vi "WriteExternalInterfaces.vi"(8 "Error In":errorcluster, 10 "ExternalInterfaces":T1[](array[typedef]), 11 "OpenCVCam in":refnum<class "OpenCVCam.lvclass">) -> (0 "Error Out":errorcluster, 3 "OpenCVCam out":refnum<class "OpenCVCam.lvclass">)   [LabVIEW 2021, in "OpenCVCam.lvclass"]
uses:
  OpenCVCam.lvclass
  .Externals/Library_TAF_Support/ClusterArrayConversion/BundledArray.ctl
  OpenCVCam.lvclass/OpenCVCam.ctl
  0f9fbe56-9f9a-4601-8b43-1fc07a995cee.vi
  0f9fbe56-9f9a-4601-8b43-1fc07a995cee.vi/e733eca7-9823-4359-8665-3b184f9a7377.vi
  0f9fbe56-9f9a-4601-8b43-1fc07a995cee.vi/185eb5ab-e8f7-4395-854b-f566a9b9020c.vi
  <vilib>/Utility/Data Type/Get Cluster Information.vi
  <vilib>/Utility/Data Type/Get Type Information.vi
  <userlib>/_OpenG.lib/lvdata/lvdata.llb/Array of VData to VCluster__ogtk.vi
  <vilib>/Utility/LVClass/Get LV Class Name.vi
  .Externals/Library_TAF_Support/ClusterArrayConversion/ClusterArrayConversion.lvlib
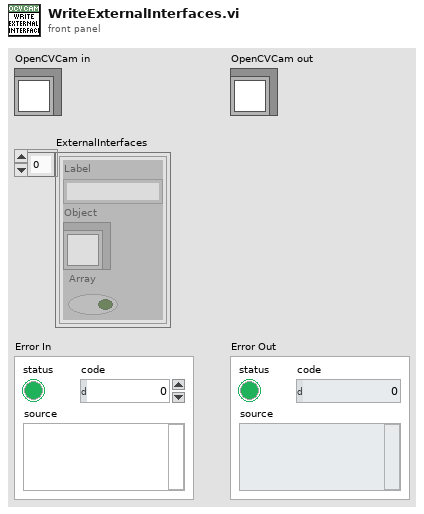
[diagram p1: front panel]
types:
  T1 = typedef "ClusterArrayConversion.lvlib/BundledArray.ctl" = cluster{"Label":string, "Object":refnum<class>, "Array":bool}
  T2 = cluster{"INewOpenCvMat":refnum<class "INewOpenCVMat.lvclass">}
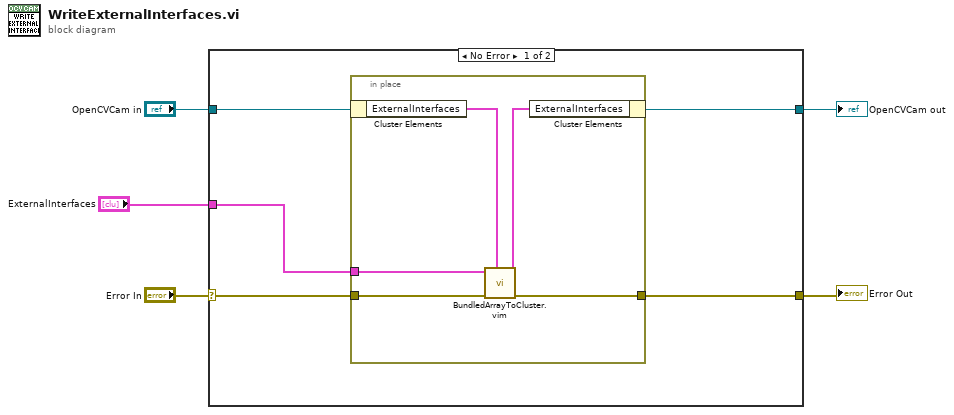
[diagram p0: block diagram]
diagram:
  n1 = case shown="No Error" "Error In" {
    selector: "Error In" -> [w8 w17]
    tunnel: [w7 w17] -> w4
    tunnel: [w9 w16] -> w2
    tunnel: "OpenCVCam in" -> [w10 w16]
    tunnel: "ExternalInterfaces" -> [w6 _]
    frame No Error {
      n2 = in-place {
        in-place-border: [w15] -> w7
        in-place-border: w8 -> [w14]
        in-place-border: w6 -> [w13]
        n3 = in-place-cluster #1(w10) -> ("ExternalInterfaces"=w12:T2)
        n4 = call "BundledArrayToCluster.vim"("Type"=w12, "error in (no error)"=w14, "BundeledLabels"=w13) -> ("error out"=w15:errorcluster, "DataOut"=w11:T2)  [unwired: 7 in]
        n5 = in-place-cluster #1("ExternalInterfaces"=w11) -> (w9:refnum<class "OpenCVCam.lvclass">)
      }
    }
    frame Error {
    }
  }
  "Error Out" <- w4
  "OpenCVCam out" <- w2
